vi "Make_Odd.vi"(1 "No of samples":i32) -> (0 "Odd No of Samples":i32)   [LabVIEW 2010]
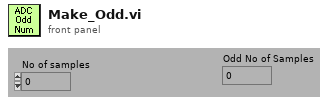
[diagram p1: front panel]
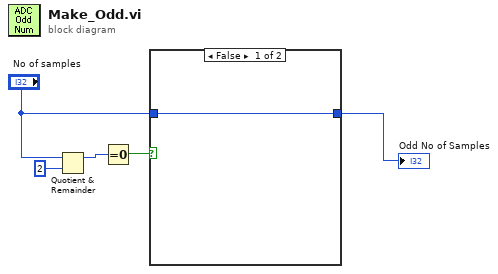
[diagram p0: block diagram]
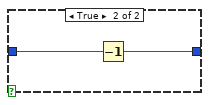
[diagram p2: hidden frame]
diagram:
  n1 = Quotient & Remainder(x="No of samples", y=2) -> (x-y*floor(x/y)=w5:i32)  [unwired: 1 out]
  n2 = Equal To 0?(x=w5) -> (x = 0?=w3:bool)
  n3 = case shown="False" w3 {
    tunnel: "No of samples" -> [w6 w8]
    tunnel: [w6 w7] -> w1
    frame False {
    }
    frame True {
      n4 = Decrement(x=w8) -> (x-1=w7:i32)
    }
  }
  "Odd No of Samples" <- w1
